vi "Stocktaking.vi"() -> ()   [LabVIEW 2019]
uses:
  <vilib>/Utility/miscctls.llb/LVMapReplaceAction.ctl
panel:
  out "Numeric":dbl
  in  "Czy jest artykuł?":string
  out "Value":dbl format="%.2f"
  out "OK Button 2":bool
  out "Ile produktów?":string
  out "Wartość":dbl format="%.2f"
  in  "STOP":bool
  in  "OK Button":bool
  in  "Artykuł":T1 {"Liczba sztuk" min=0.0 format="%#1_6g"; "Cena za sztukę" format="%.2f"}
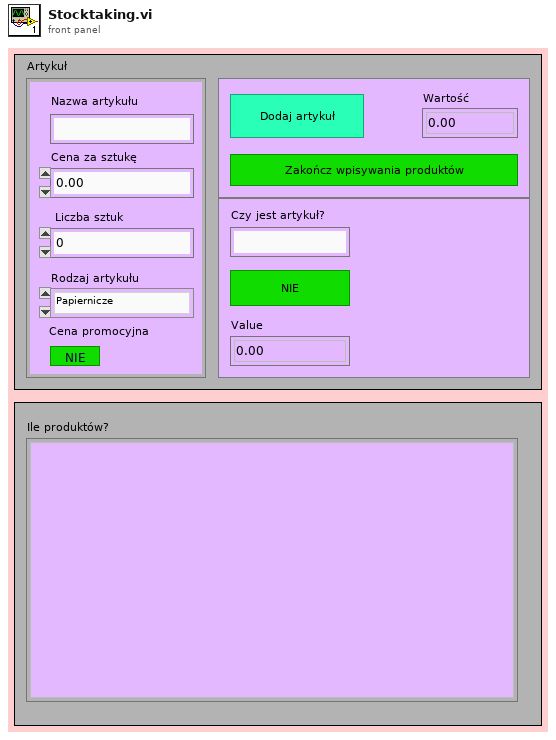
[diagram p1: front panel]
types:
  T1 = cluster{"Nazwa artykułu":string, "Cena za sztukę":dbl, " Liczba sztuk":dbl, "Rodzaj artykułu":enum16{"Papiernicze", "Kosmetyki", "Spożywcze", "Chemia gospodarcza"}, "Cena promocyjna":bool}
  T2 = map{enum16{"Papiernicze", "Kosmetyki", "Spożywcze", "Chemia gospodarcza"}, i32}
  T3 = typedef "LVMapReplaceAction.ctl" = enum32{"Modify Entry only if found", "Add or Modify Entry", "Delete Entry"}
  T4 = enum16{"Papiernicze", "Kosmetyki", "Spożywcze", "Chemia gospodarcza"}
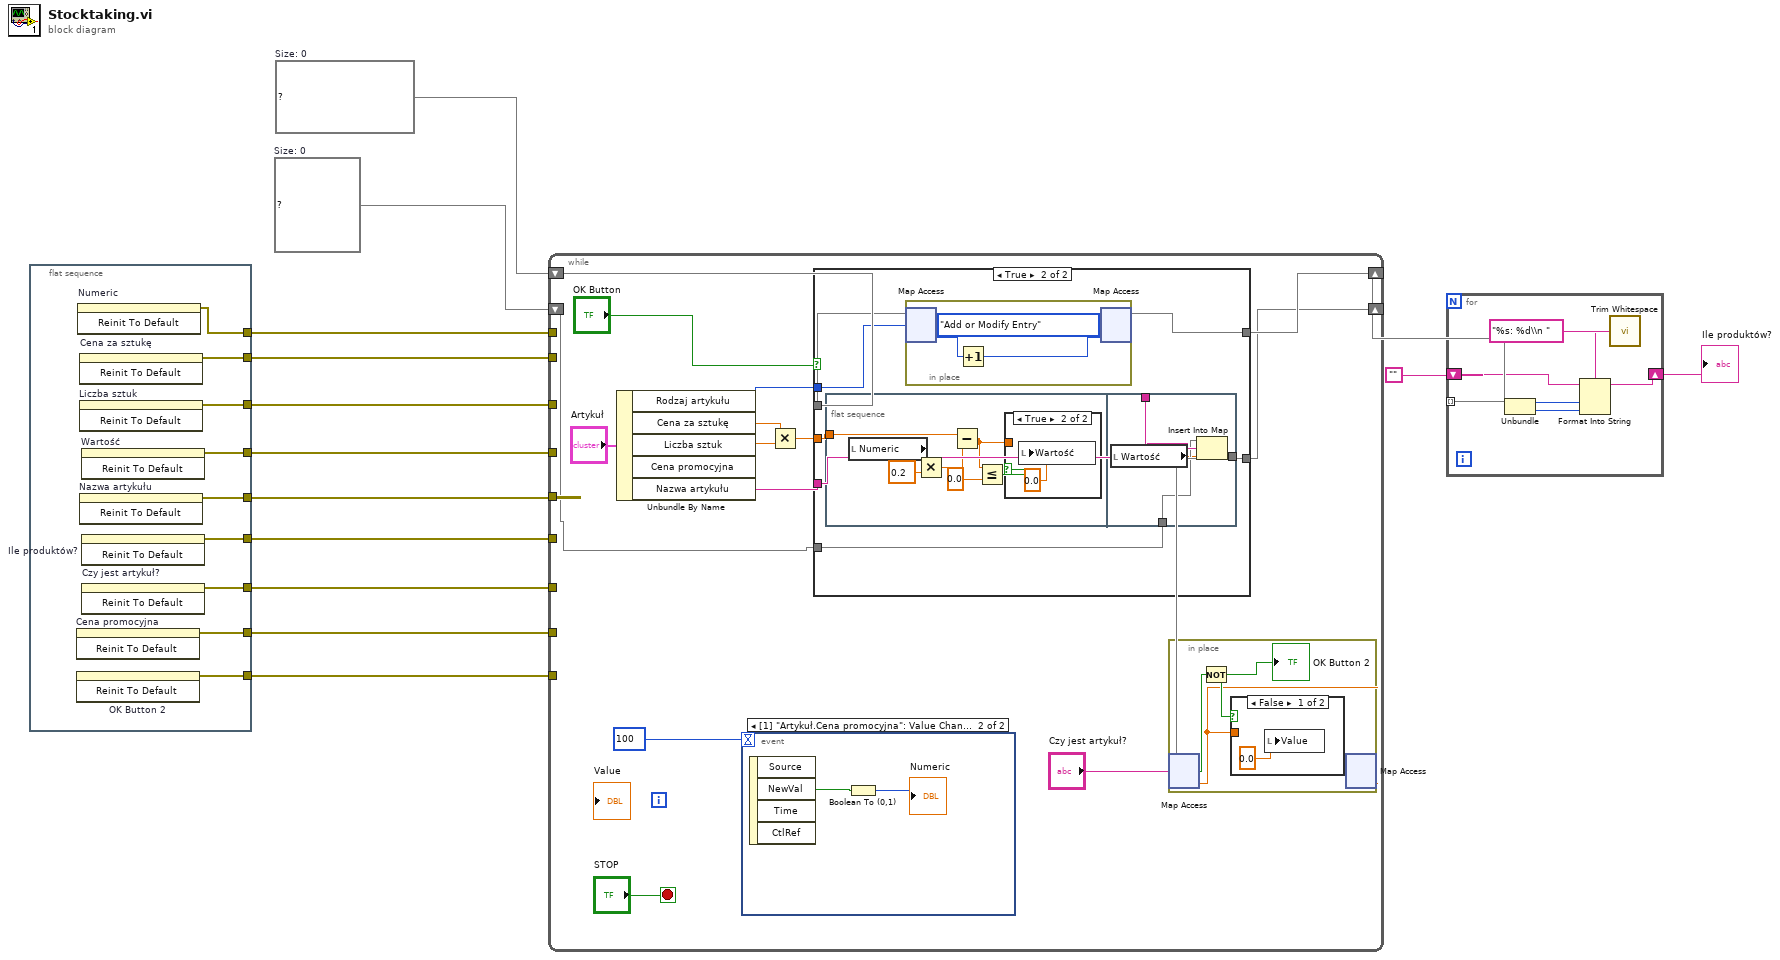
[diagram p0: block diagram]
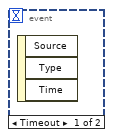
[diagram p2: hidden frame]
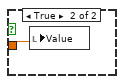
[diagram p3: hidden frame]
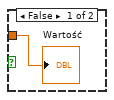
[diagram p5: hidden frame]
diagram:
  w10 = map{string, dbl} {}  # Size: 0
  w11 = T2 {}  # Size: 0
  n1 = flat-sequence {
    tunnel: [w23] -> w9
    tunnel: [w22] -> w8
    tunnel: [w21] -> w7
    tunnel: [w20] -> w6
    tunnel: [w19] -> w5
    tunnel: [w18] -> w4
    tunnel: [w17] -> w3
    tunnel: [w16] -> w2
    tunnel: [w15] -> w1
    frame #0 {
      n2 = invoke on="Cena promocyjna" class="Bool (strict)" method="Reinit To Default"() -> (error out=w16:errorcluster)  [unwired: 3 in, 2 out]
      n3 = invoke on="OK Button 2" class="Bool" method="Reinit To Default"() -> (error out=w15:errorcluster)  [unwired: 3 in, 2 out]
      n4 = invoke on="Numeric" class="DigNum (strict)" method="Reinit To Default"() -> (error out=w23:errorcluster)  [unwired: 3 in, 2 out]
      n5 = invoke on="Cena za sztukę" class="DigNum (strict)" method="Reinit To Default"() -> (error out=w22:errorcluster)  [unwired: 3 in, 2 out]
      n6 = invoke on="Liczba sztuk" class="DigNum (strict)" method="Reinit To Default"() -> (error out=w21:errorcluster)  [unwired: 3 in, 2 out]
      n7 = invoke on="Nazwa artykułu" class="Str" method="Reinit To Default"() -> (error out=w19:errorcluster)  [unwired: 3 in, 2 out]
      n8 = invoke on="Wartość" class="DigNum (strict)" method="Reinit To Default"() -> (error out=w20:errorcluster)  [unwired: 3 in, 2 out]
      n9 = invoke on="Ile produktów?" class="Str" method="Reinit To Default"() -> (error out=w18:errorcluster)  [unwired: 3 in, 2 out]
      n10 = invoke on="Czy jest artykuł?" class="Str" method="Reinit To Default"() -> (error out=w17:errorcluster)  [unwired: 3 in, 2 out]
    }
  }
  n11 = while {
    shift-right: [w31] -> w14
    shift-left: w11 -> [w32]
    shift-right: [w26] -> _
    shift-left: w10 -> [w24]
    tunnel: w9 -> [_]
    tunnel: w8 -> [_]
    tunnel: w7 -> [_]
    tunnel: w6 -> [_]
    tunnel: w5 -> [_]
    tunnel: w4 -> [_]
    tunnel: w3 -> [_]
    tunnel: w2 -> [_]
    tunnel: w1 -> [_]
    stop <- "STOP" stop-if-true
    n12 = Unbundle By Name("Artykuł") -> ("Rodzaj artykułu"=w28:T4, "Cena za sztukę"=w34:dbl, "Liczba sztuk"=w35:dbl, "Nazwa artykułu"=w29:string)  [unwired: 1 out]
    n13 = event shown="[1] \"Artykuł.Cena promocyjna\": Value Change" {
      selector: _ -> [_ _]
      dyn-events: _ -> [_ _]
      timeout: 100 -> [_ _]
      event Timeout {
        n14 = event-data() -> ()  [unwired: 1 in, 3 out]
      }
      event "Artykuł.Cena promocyjna": Value Change {
        n15 = event-data() -> ("NewVal"=w39:bool)  [unwired: 1 in, 3 out]
        n16 = Boolean To (0,1)(Boolean=w39) -> (0, 1=→"Numeric":i16)
      }
    }
    n17 = Multiply(x=w34, y=w35) -> (x*y=w33:dbl)
    n18 = case shown="True" "OK Button" {
      tunnel: w33 -> [_ w50]
      tunnel: w32 -> [w46 w53]
      tunnel: [w46 w52] -> w31
      tunnel: [w45 w48] -> w26
      tunnel: w29 -> [_ w49]
      tunnel: w28 -> [_ w51]
      tunnel: w24 -> [w45 w47]
      frame False {
      }
      frame True {
        n19 = flat-sequence {
          tunnel: w50 -> [w60]
          tunnel: w49 -> [w66]
          tunnel: w47 -> [w65]
          tunnel: [w64] -> w48
          frame #0 {
            n20 = local read "Numeric"() -> (w58:dbl)
            n21 = Multiply(x=w58, y=0.2) -> (x*y=w59:dbl)
            n22 = Subtract(x=w60, y=w59) -> (x-y=w54:dbl)
            n23 = Less Or Equal?(x=w54, y=0.0) -> (x <= y?=w55:bool)
            n24 = case shown="True" w55 {
              tunnel: w54 -> [w61 _]
              frame False {
                "Wartość" <- w61
              }
              frame True {
                n25 = local write "Wartość"(0.0 ("wartość")) -> ()
              }
            }
          }
          frame #1 {
            n26 = local read "Wartość"() -> (w63:dbl)
            n27 = Insert Into Map(map in=w65, key=w66, value=w63) -> (map out=w64:map{string, dbl})  [unwired: 2 out]
          }
        }
        n28 = in-place {
          n29 = in-place-map #1(w53, w51) -> (w68:i32)  [unwired: 1 in, 1 out]
          n30 = Increment(x=w68) -> (x+1=w67:i32)
          n31 = in-place-map #1(w67, LVMapReplaceAction."Add or Modify Entry" ("action")) -> (w52:T2)  [unwired: 2 out]
        }
      }
    }
    n32 = in-place {
      n33 = in-place-map #2(w26, "Czy jest artykuł?") -> (w40:dbl, w42:bool)  [unwired: 1 in]
      n34 = Not(x=w42) -> (.not. x?=w41:bool)
      "OK Button 2" <- w41
      n35 = case shown="False" w41 {
        tunnel: w40 -> [_ w44]
        frame False {
          n36 = local write "Value"(0.0 ("value")) -> ()
        }
        frame True {
          n37 = local write "Value"(w44) -> ()
        }
      }
      n38 = in-place-map #2(w40) -> ()  [unwired: 1 in, 3 out]
    }
  }
  n39 = for {
    tunnel: w14 -> [w76] mode=indexing
    shift-right: [w72] -> w12
    shift-left: "" -> [w73]
    n40 = Unbundle(w76) -> ("Rodzaj artykułu"=w74:T4, w75:i32)
    n41 = call <vilib>:"Trim Whitespace.vi"("string"="%s: %d\\n " ("format string")) -> ("trimmed string"=w70:string)  [unwired: 1 in]
    n42 = Format Into String(format string=w70, initial string=w73, w74, w75) -> (resulting string=w72:string)  [unwired: 1 in, 1 out]
  }
  "Ile produktów?" <- w12
